vi "power conversions.vi"(10 "Current Raw":dbl, 11 "Voltage Raw":dbl) -> (2 "Current":dbl, 3 "Voltage":dbl)   [LabVIEW 2014]
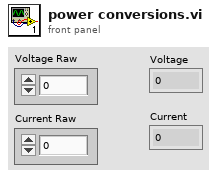
[diagram p1: front panel]
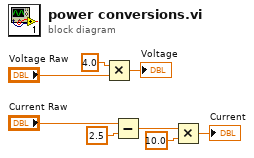
[diagram p0: block diagram]
diagram:
  n1 = Multiply(x=4.0, y="Voltage Raw") -> (x*y=→"Voltage":dbl)
  n2 = Subtract(x="Current Raw", y=2.5) -> (x-y=w5:dbl)
  n3 = Multiply(x=w5, y=10.0) -> (x*y=→"Current":dbl)
